vi "SetMode.vi"(8 "error in (no error)":errorcluster, 10 "Mode":T1, 11 "ScopeBase In":refnum<class "ScopeBase.lvclass">) -> (0 "error out":errorcluster, 3 "ScopeBase Out":refnum<class "ScopeBase.lvclass">)   [LabVIEW 2018, in "ScopeBase.lvclass"]
uses:
  ScopeBase.lvclass
  FPGA/DataMode.ctl
  ScopeBase.lvclass/ScopeBase.ctl
  <vilib>/Utility/error.llb/Error Cluster From Error Code.vi
  <vilib>/rvi/errors/niLvFpgaAdjustHostInterfaceError.vi
  <vilib>/rvi/interface/nirviReadWriteControl/nirviReadWriteControl.xnode
  FpgaRef/FpgaRefBase/Common FPGA ref.ctl
  FpgaRef/FpgaRefBase/FpgaRefBase.lvclass
  NiFpgaLv.dll
  <vilib>/rvi/interface/Simulation/niFpgaSimulationCallBeginRW.vi
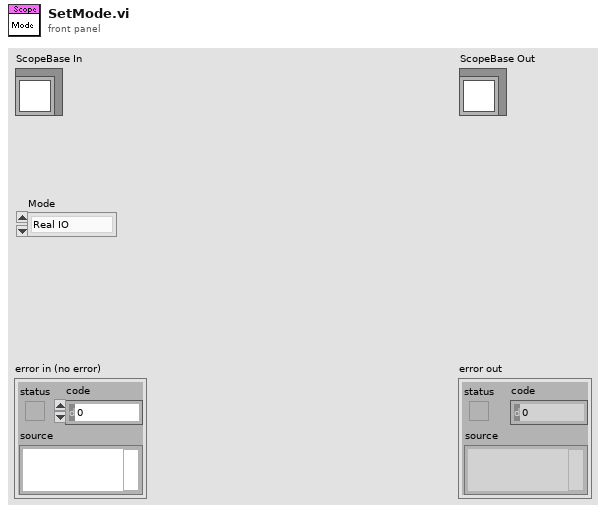
[diagram p1: front panel]
types:
  T1 = typedef "DataMode.ctl" = enum16{"Real IO", "Simulated"}
  T2 = typedef "Common FPGA ref.ctl" = refnum<k20>
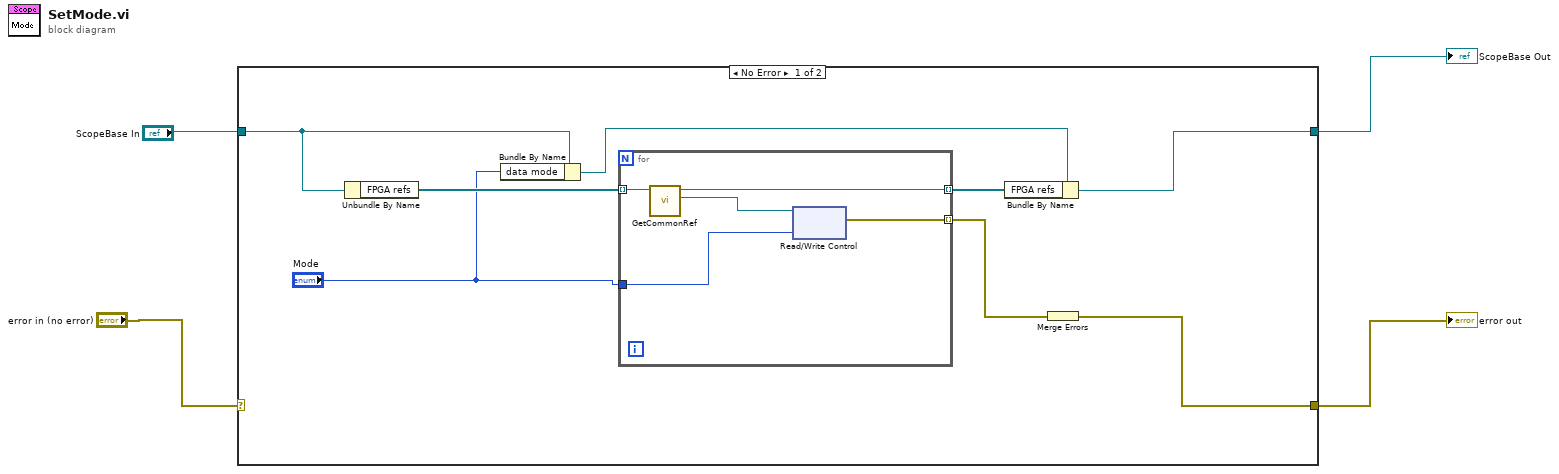
[diagram p0: block diagram]
diagram:
  n1 = case shown="No Error" "error in (no error)" {
    selector: "error in (no error)" -> [_ w19]
    tunnel: [w5 w19] -> w1
    tunnel: [w10 w18] -> w2
    tunnel: "ScopeBase In" -> [w9 w18]
    frame No Error {
      n2 = Unbundle By Name(w9) -> ("FPGA refs"=w12:refnum<class "FpgaRefBase.lvclass">[])
      n3 = Bundle By Name(cluster=w9, "data mode"="Mode") -> (w8:refnum<class "ScopeBase.lvclass">)
      n4 = for {
        tunnel: "Mode" -> [w14]
        tunnel: w12 -> [w17] mode=indexing
        tunnel: [w16] -> w11 mode=indexing
        tunnel: [w13] -> w6 mode=indexing
        n5 = call-dynamic "GetCommonRef.vi"("FpgaRefBase in"=w17) -> ("Common ref"=w15:T2, "FpgaRefBase out"=w16:refnum<class "FpgaRefBase.lvclass">)  [unwired: 8 in, 1 out]
        n6 = xnode "Read/Write Control"("FPGA VI Reference In"=w15, "Mode"=w14) -> ("error out"=w13:errorcluster)  [unwired: 1 in, 1 out]
      }
      n7 = Bundle By Name(cluster=w8, "FPGA refs"=w11) -> (w10:refnum<class "ScopeBase.lvclass">)
      n8 = Merge Errors(w6) -> (w5:errorcluster)
    }
    frame Error {
    }
  }
  "error out" <- w1
  "ScopeBase Out" <- w2
